vi "UE_C_LV2.vi"(0 "Event_Data":T1={"Event_Data"=0.0, "PlayBack?"=TRUE}, 11 "Error_In":errorcluster, 13 "Operation":T2=enum."Get_UE_Reference") -> (4 "Event_Reference":refnum<event-registration>, 15 "Error_Out":errorcluster)   [LabVIEW 2021]
doc: "Used to Create, generate and destroy the user event."
uses:
  Controls/Operation.ctl
  Controls/Event_Data.ctl
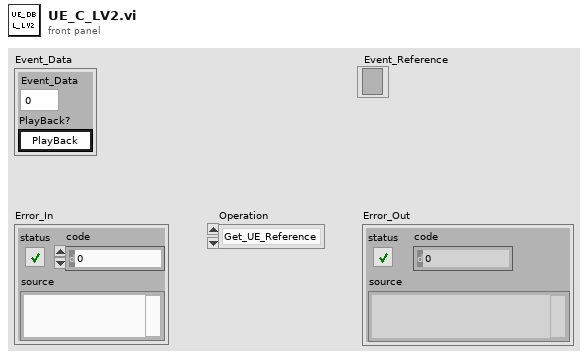
[diagram p1: front panel]
types:
  T1 = typedef "Event_Data.ctl" = cluster{"Event_Data":dbl, "PlayBack?":bool}
  T2 = typedef "Operation.ctl" = enum16{"Create_UE", "Generate_UE", "Destroy_UE", "Get_UE_Reference"}
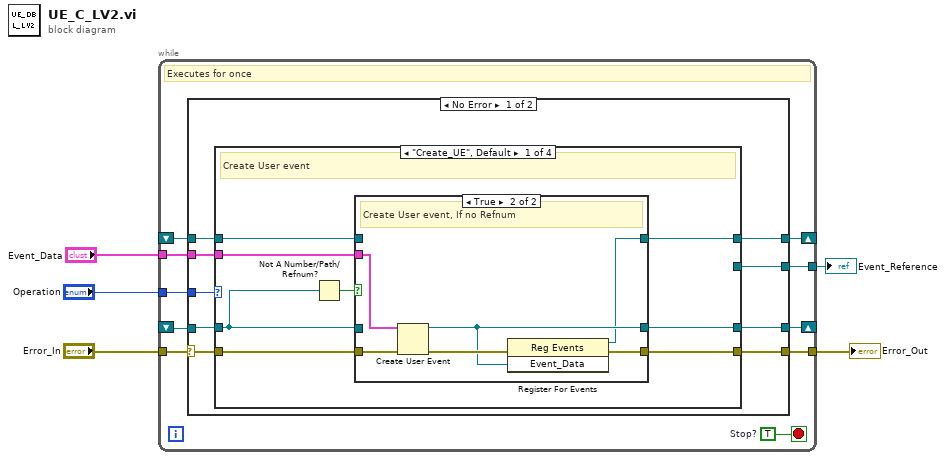
[diagram p0: block diagram]
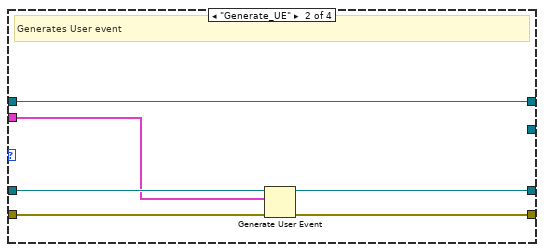
[diagram p3: hidden frame]
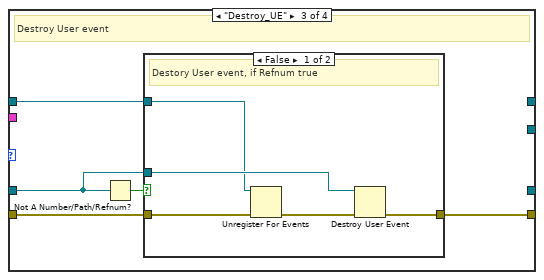
[diagram p4: hidden frame]
diagram:
  n1 = while {
    tunnel: "Error_In" -> [w15]
    shift-right: [w12] -> _
    shift-left: _ -> [w11]
    tunnel: "Operation" -> [w14]
    tunnel: [w13] -> w3
    tunnel: "Event_Data" -> [w10]
    shift-right: [w8] -> _
    shift-left: _ -> [w7]
    tunnel: [w6] -> w1
    stop <- w9 stop-if-true
    w9 = TRUE  # Stop?
    # "Executes for once"
    n2 = case shown="No Error" w15 {
      selector: w15 -> [w23 w64]
      tunnel: w14 -> [w24 _]
      tunnel: [w22 w64] -> w13
      tunnel: [w21 w63] -> w12
      tunnel: w11 -> [w19 w63]
      tunnel: w10 -> [w20 _]
      tunnel: [w18 w62] -> w8
      tunnel: w7 -> [w17 w62]
      tunnel: [w16 _] -> w6
      frame No Error {
        n3 = case shown="\"Create_UE\", Default" w24 {
          tunnel: w23 -> [w32 w47 w52 w60]
          tunnel: [w31 w46 w51 w60] -> w22
          tunnel: [w30 w45 _ w61] -> w21
          tunnel: w20 -> [w28 w43 _ _]
          tunnel: w19 -> [w27 w44 w49 w61]
          tunnel: [w26 w42 _ w59] -> w18
          tunnel: w17 -> [w25 w42 w48 w59]
          tunnel: [_ _ _ w59] -> w16
          frame "Create_UE", Default {
            # "Create User event"
            n4 = Not A Number/Path/Refnum?(number/path/refnum=w27) -> (NaN/Path/Refnum?=w29:bool)
            n5 = case shown="True" w29 {
              tunnel: w32 -> [w34 w41]
              tunnel: [w34 w38] -> w31
              tunnel: [w35 w37] -> w30
              tunnel: w27 -> [w35 _]
              tunnel: w28 -> [_ w39]
              tunnel: [w33 w36] -> w26
              tunnel: w25 -> [w33 _]
              frame False {
              }
              frame True {
                # "Create User event, If no Refnum"
                n6 = Create User Event(user event datatype=w39, error in=w41) -> (user event=w37:refnum<user-event>, error out=w40:errorcluster)
                n7 = register-events(error in=w40, w37) -> (reference out=w36:refnum<event-registration>, error out=w38:errorcluster)  [unwired: 1 in]
              }
            }
          }
          frame "Generate_UE" {
            # "Generates User event"
            n8 = Generate User Event(user event=w44, event data cluster=w43, error in=w47) -> (user event out=w45:refnum<user-event>, error out=w46:errorcluster)  [unwired: 1 in]
          }
          frame "Destroy_UE" {
            # "Destroy User event"
            n9 = Not A Number/Path/Refnum?(number/path/refnum=w49) -> (NaN/Path/Refnum?=w50:bool)
            n10 = case shown="False" w50 {
              tunnel: w52 -> [w55 w58]
              tunnel: [w57 w58] -> w51
              tunnel: w49 -> [w56 _]
              tunnel: w48 -> [w53 _]
              frame False {
                # "Destory User event, if Refnum true"
                n11 = Unregister For Events(event registration refnum=w53, error in=w55) -> (error out=w54:errorcluster)
                n12 = Destroy User Event(user event=w56, error in=w54) -> (error out=w57:errorcluster)
              }
              frame True {
              }
            }
          }
          frame "Get_UE_Reference" {
            # "Returns out Refnum of the User event"
          }
        }
      }
      frame Error {
      }
    }
  }
  "Error_Out" <- w3
  "Event_Reference" <- w1
